vi "Form VTG Sentence.vi"(8 "error in (no error)":errorcluster, 11 "VTG  data":T1={"true track made good"={"included?"=TRUE, "true track made good (deg)"=0.0}, "magnetic track made good"={"included?"=TRUE, "magnetic track made good (deg)"=0.0}, "ground speed (knots)"={"included?"=TRUE, "speed (knots)"=0.0}, "ground speed (km/h)"={"included?"=TRUE, "speed (km/h)"=0.0}, "type of fix"={"included?"=TRUE, "mode"=0}} {"type of fix"."mode" items=["", "Simulator", "Not Valid", "Estimated", "Differential", "Autonomous"]}) -> (0 "error out":errorcluster, 3 "VTG sentence":string)   [LabVIEW 2009]
doc: "Creates an NMEA sentence using the data you specify for a particular sentence type. You must manually select the polymorphic instance to use."
uses:
  typedefs/VTG Data.ctl
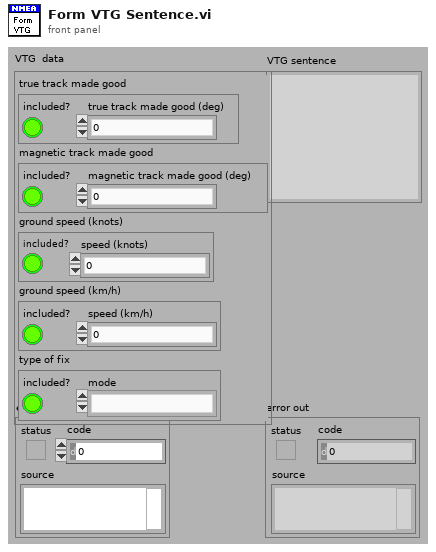
[diagram p1: front panel]
types:
  T1 = typedef "VTG Data.ctl" = cluster{"true track made good":cluster{"included?":bool, "true track made good (deg)":dbl}, "magnetic track made good":cluster{"included?":bool, "magnetic track made good (deg)":dbl}, "ground speed (knots)":cluster{"included?":bool, "speed (knots)":dbl}, "ground speed (km/h)":cluster{"included?":bool, "speed (km/h)":dbl}, "type of fix":cluster{"included?":bool, "mode":u16}}
  T2 = cluster{"included?":bool, "true track made good (deg)":dbl}
  T3 = cluster{"included?":bool, "magnetic track made good (deg)":dbl}
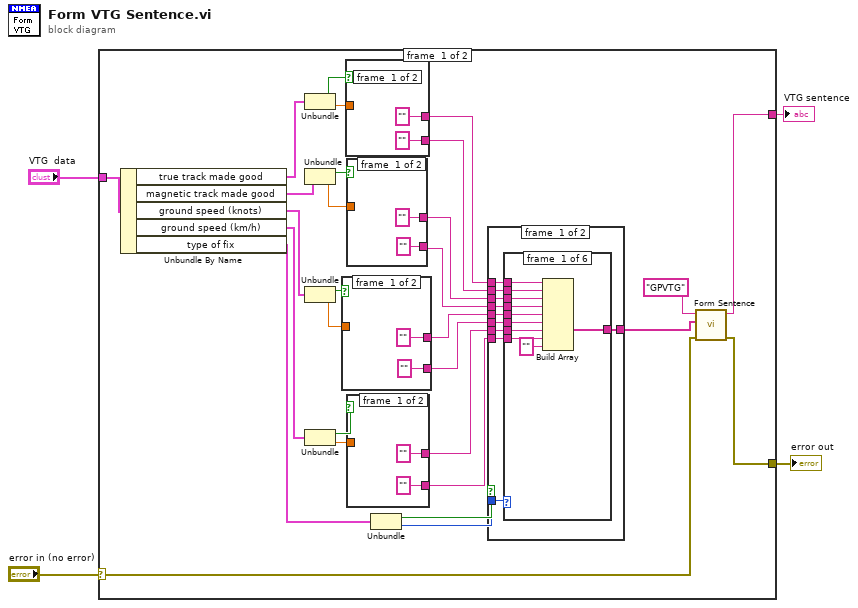
[diagram p0: block diagram]
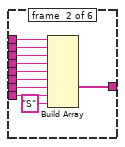
[diagram p2: hidden frame]
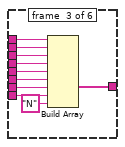
[diagram p3: hidden frame]
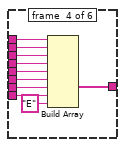
[diagram p4: hidden frame]
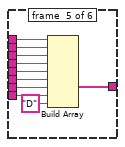
[diagram p5: hidden frame]
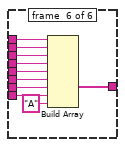
[diagram p6: hidden frame]
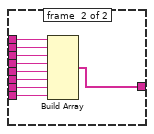
[diagram p7: hidden frame]
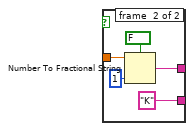
[diagram p8: hidden frame]
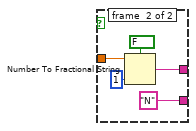
[diagram p9: hidden frame]
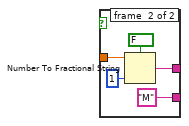
[diagram p10: hidden frame]
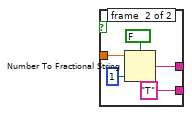
[diagram p11: hidden frame]
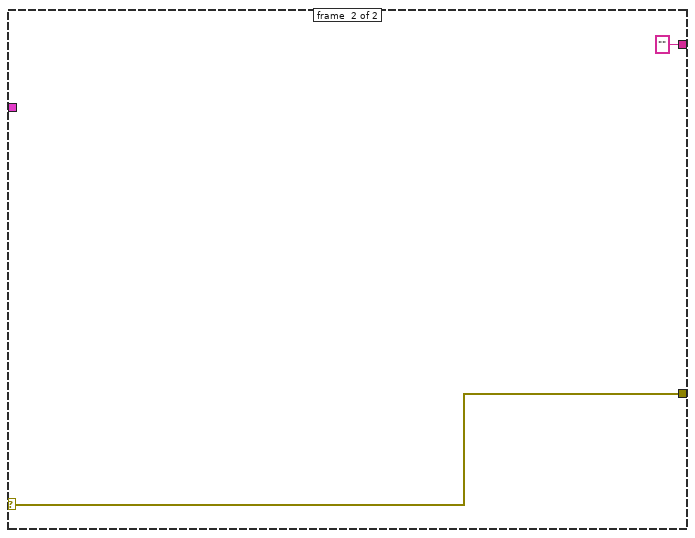
[diagram p12: hidden frame]
diagram:
  n1 = case shown="No Error" "error in (no error)" {
    selector: "error in (no error)" -> [w30 w141]
    tunnel: "VTG  data" -> [w33 _]
    tunnel: [w29 w141] -> w2
    tunnel: [w28 "" ("NMEA Sentence")] -> w1
    frame #0 {
      n2 = Unbundle By Name(w33) -> ("true track made good"=w22:T2, "magnetic track made good"=w21:T3, "ground speed (knots)"=w17:cluster{"included?":bool, "speed (knots)":dbl}, "ground speed (km/h)"=w18:cluster{"included?":bool, "speed (km/h)":dbl}, "type of fix"=w7:cluster{"included?":bool, "mode":u16})
      n3 = Unbundle(w22) -> ("included?"=w15:bool, "true track made good (deg)"=w23:dbl)
      n4 = Unbundle(w21) -> ("included?"=w14:bool, "magnetic track made good (deg)"=w20:dbl)
      n5 = Unbundle(w17) -> ("included?"=w13:bool, "speed (knots)"=w16:dbl)
      n6 = Unbundle(w18) -> ("included?"=w12:bool, "speed (km/h)"=w19:dbl)
      n7 = case shown="True" w13 {
        tunnel: ["" w126] -> w25
        tunnel: w16 -> [_ w125]
        tunnel: ["" ("element") "N" ("element")] -> w9
        frame #0 {
        }
        frame #1 {
          n8 = Number To Fractional String(use system decimal point (T)=FALSE, number=w125, precision (6)=i16 1) -> (F-format string=w126:string)  [unwired: 1 out]
        }
      }
      n9 = case shown="True" w15 {
        tunnel: ["" w140] -> w27
        tunnel: w23 -> [_ w139]
        tunnel: ["" ("element") "T" ("element")] -> w11
        frame #0 {
        }
        frame #1 {
          n10 = Number To Fractional String(use system decimal point (T)=FALSE, number=w139, precision (6)=i16 1) -> (F-format string=w140:string)  [unwired: 1 out]
        }
      }
      n11 = case shown="True" w14 {
        tunnel: ["" w133] -> w26
        tunnel: w20 -> [_ w132]
        tunnel: ["" ("element") "M" ("element")] -> w10
        frame #0 {
        }
        frame #1 {
          n12 = Number To Fractional String(use system decimal point (T)=FALSE, number=w132, precision (6)=i16 1) -> (F-format string=w133:string)  [unwired: 1 out]
        }
      }
      n13 = case shown="True" w12 {
        tunnel: ["" w119] -> w24
        tunnel: w19 -> [_ w118]
        tunnel: ["" ("element") "K" ("element")] -> w8
        frame #0 {
        }
        frame #1 {
          n14 = Number To Fractional String(use system decimal point (T)=FALSE, number=w118, precision (6)=i16 1) -> (F-format string=w119:string)  [unwired: 1 out]
        }
      }
      n15 = Unbundle(w7) -> ("included?"=w6:bool, "mode"=w5:u16)
      n16 = case shown="True" w6 {
        tunnel: [w43 w112] -> w31
        tunnel: w27 -> [w42 w111]
        tunnel: w26 -> [w41 w110]
        tunnel: w25 -> [w40 w109]
        tunnel: w24 -> [w39 w108]
        tunnel: w11 -> [w38 w107]
        tunnel: w10 -> [w37 w106]
        tunnel: w9 -> [w36 w105]
        tunnel: w8 -> [w35 w104]
        tunnel: w5 -> [w34 _]
        frame #0 {
          n17 = case shown="Default" w34 {
            tunnel: [w53 w63 w73 w83 w93 w103] -> w43
            tunnel: w42 -> [w52 w62 w72 w82 w92 w102]
            tunnel: w41 -> [w51 w61 w71 w81 w91 w101]
            tunnel: w40 -> [w50 w60 w70 w80 w90 w100]
            tunnel: w39 -> [w49 w59 w69 w79 w89 w99]
            tunnel: w38 -> [w48 w58 w68 w78 w88 w98]
            tunnel: w37 -> [w47 w57 w67 w77 w87 w97]
            tunnel: w36 -> [w46 w56 w66 w76 w86 w96]
            tunnel: w35 -> [w45 w55 w65 w75 w85 w95]
            frame #0 {
              n18 = Build Array(w52, w48, w51, w47, w50, w46, w49, w45, "" ("element")) -> (w53:string[])
            }
            frame #1 {
              n19 = Build Array(w62, w58, w61, w57, w60, w56, w59, w55, "S" ("element")) -> (w63:string[])
            }
            frame #2 {
              n20 = Build Array(w72, w68, w71, w67, w70, w66, w69, w65, "N" ("element")) -> (w73:string[])
            }
            frame #3 {
              n21 = Build Array(w82, w78, w81, w77, w80, w76, w79, w75, "E" ("element")) -> (w83:string[])
            }
            frame #4 {
              n22 = Build Array(w92, w88, w91, w87, w90, w86, w89, w85, "D" ("element")) -> (w93:string[])
            }
            frame #5 {
              n23 = Build Array(w102, w98, w101, w97, w100, w96, w99, w95, "A" ("element")) -> (w103:string[])
            }
          }
        }
        frame #1 {
          n24 = Build Array(w111, w107, w110, w106, w109, w105, w108, w104) -> (w112:string[])
        }
      }
      n25 = call "Form Sentence.vi"("error in (no error)"=w30, "sentence data"=w31, "sentence type"="GPVTG" ("Sentence Type")) -> ("error out"=w29:errorcluster, "sentence"=w28:string)  [unwired: 5 in]
    }
    frame #1 {
    }
  }
  "error out" <- w2
  "VTG sentence" <- w1
